vi "VI Tree.vi"   [LabVIEW 2011, in "Agilent PSG MXG Series.lvlib"]
doc: "This is the instrument driver for the Agilent PSG MXG Series. The VI Tree displays all the user-callable VIs of the instrument driver in an organized table."
uses:
  Agilent PSG MXG Series.lvlib
  Configure/Configure Sweep (List).vi
  Configure/Modulation/Configure Modulation (Amplitude).vi
  Configure/Modulation/Configure Modulation Waveform (Noise).vi
panel:
  # "(c) 2011 National Instruments.  ALL RIGHTS RESERVED."
  # "SEE DIAGRAM\nFOR VI TREE."
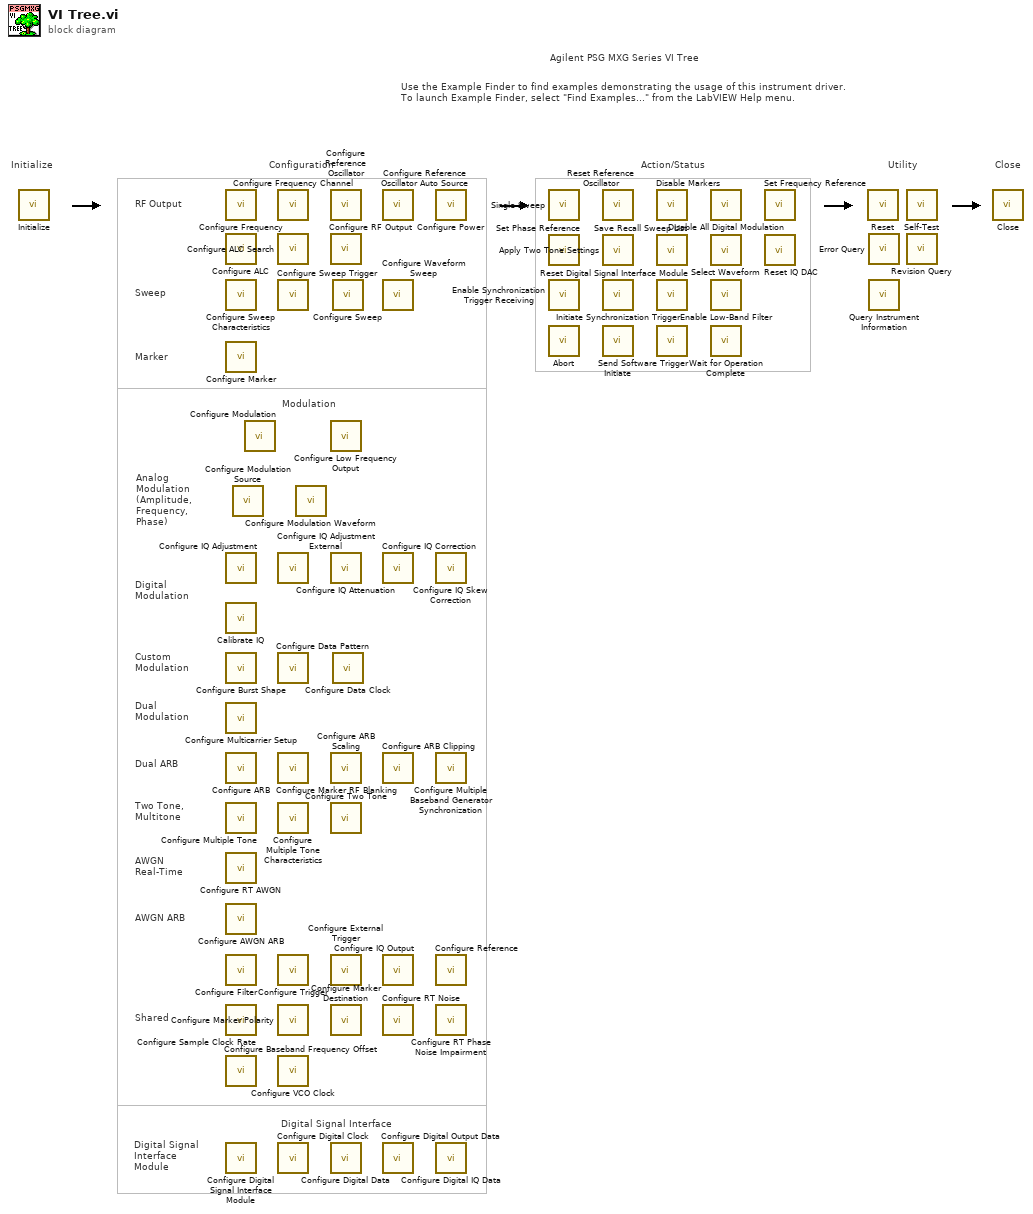
[diagram p0: block diagram]
diagram:
  # "AWGN ARB"
  # "Digital Signal Interface"
  # "Marker"
  # "Digital Signal\nInterface\nModule"
  # "AWGN\nReal-Time"
  # "Shared"
  # "Two Tone,\nMultitone"
  # "Dual ARB"
  # "Dual\nModulation"
  # "Custom\nModulation"
  # "Digital\nModulation"
  # "Analog\nModulation\n(Amplitude,\nFrequency,\nPhase)"
  # "Sweep"
  # "RF Output"
  # "Modulation"
  # "Agilent PSG MXG Series VI Tree"
  # "Use the Example Finder to find examples demonstrating the usage of this instrument driver.\nTo launch Example Finder, select \"Find Examples...\" from the LabVIEW Help menu."
  # "Configuration"
  # "Utility"
  # "Action/Status"
  # "Close"
  # "Initialize"
  n1 = call "Initialize.vi"() -> ()  [unwired: 10 in, 2 out]
  n2 = call "Configure Frequency.vi"() -> ()  [unwired: 14 in, 2 out]
  n3 = call "Configure ALC.vi"() -> ()  [unwired: 14 in, 2 out]
  n4 = call "Configure Sweep Characteristics.vi"() -> ()  [unwired: 14 in, 2 out]
  n5 = call "Configure Marker.vi"() -> ()  [unwired: 14 in, 2 out]
  n6 = call "Configure IQ Adjustment.vi"() -> ()  [unwired: 14 in, 2 out]
  n7 = call "Calibrate IQ.vi"() -> ()  [unwired: 10 in, 2 out]
  n8 = call "Configure Burst Shape.vi"() -> ()  [unwired: 14 in, 2 out]
  n9 = call "Configure Multicarrier Setup.vi"() -> ()  [unwired: 14 in, 2 out]
  n10 = call "Configure ARB.vi"() -> ()  [unwired: 10 in, 2 out]
  n11 = call "Configure Multiple Tone.vi"() -> ()  [unwired: 14 in, 2 out]
  n12 = call "Configure RT AWGN.vi"() -> ()  [unwired: 10 in, 2 out]
  n13 = call "Configure AWGN ARB.vi"() -> ()  [unwired: 10 in, 2 out]
  n14 = call "Configure Filter.vi"() -> ()  [unwired: 14 in, 2 out]
  n15 = call "Configure Sample Clock Rate.vi"() -> ()  [unwired: 10 in, 2 out]
  n16 = call "Configure Baseband Frequency Offset.vi"() -> ()  [unwired: 10 in, 2 out]
  n17 = call "Configure Digital Signal Interface Module.vi"() -> ()  [unwired: 10 in, 2 out]
  n18 = call "Configure Modulation Source.vi"() -> ()  [unwired: 14 in, 2 out]
  n19 = call-poly "Configure Modulation.vi"() -> ()  [unwired: 14 in, 2 out]
  n20 = call "Configure Frequency Channel.vi"() -> ()  [unwired: 10 in, 2 out]
  n21 = call "Configure ALC Search.vi"() -> ()  [unwired: 14 in, 2 out]
  n22 = call "Configure Sweep Trigger.vi"() -> ()  [unwired: 14 in, 2 out]
  n23 = call "Configure IQ Adjustment External.vi"() -> ()  [unwired: 14 in, 2 out]
  n24 = call "Configure Data Pattern.vi"() -> ()  [unwired: 10 in, 2 out]
  n25 = call "Configure Marker RF Blanking.vi"() -> ()  [unwired: 10 in, 2 out]
  n26 = call "Configure Multiple Tone Characteristics.vi"() -> ()  [unwired: 10 in, 2 out]
  n27 = call "Configure Trigger.vi"() -> ()  [unwired: 14 in, 2 out]
  n28 = call "Configure Marker Polarity.vi"() -> ()  [unwired: 10 in, 2 out]
  n29 = call "Configure VCO Clock.vi"() -> ()  [unwired: 10 in, 2 out]
  n30 = call "Configure Digital Clock.vi"() -> ()  [unwired: 14 in, 2 out]
  n31 = call-poly "Configure Modulation Waveform.vi"() -> ()  [unwired: 10 in, 2 out]
  n32 = call "Configure Reference Oscillator.vi"() -> ()  [unwired: 10 in, 2 out]
  n33 = call "Configure RF Output.vi"() -> ()  [unwired: 10 in, 2 out]
  n34 = call "Configure Low Frequency Output.vi"() -> ()  [unwired: 14 in, 2 out]
  n35 = call "Configure IQ Attenuation.vi"() -> ()  [unwired: 10 in, 2 out]
  n36 = call "Configure ARB Scaling.vi"() -> ()  [unwired: 10 in, 2 out]
  n37 = call "Configure Two Tone.vi"() -> ()  [unwired: 10 in, 2 out]
  n38 = call "Configure External Trigger.vi"() -> ()  [unwired: 10 in, 2 out]
  n39 = call "Configure Marker Destination.vi"() -> ()  [unwired: 10 in, 2 out]
  n40 = call "Configure Digital Data.vi"() -> ()  [unwired: 14 in, 2 out]
  n41 = call-poly "Configure Sweep.vi"() -> ()  [unwired: 14 in, 2 out]
  n42 = call "Configure Data Clock.vi"() -> ()  [unwired: 10 in, 2 out]
  n43 = call "Configure Reference Oscillator Auto Source.vi"() -> ()  [unwired: 10 in, 2 out]
  n44 = call "Configure Waveform Sweep.vi"() -> ()  [unwired: 10 in, 2 out]
  n45 = call "Configure IQ Correction.vi"() -> ()  [unwired: 10 in, 2 out]
  n46 = call "Configure ARB Clipping.vi"() -> ()  [unwired: 10 in, 2 out]
  n47 = call "Configure IQ Output.vi"() -> ()  [unwired: 14 in, 2 out]
  n48 = call "Configure RT Noise.vi"() -> ()  [unwired: 14 in, 2 out]
  n49 = call "Configure Digital Output Data.vi"() -> ()  [unwired: 10 in, 2 out]
  n50 = call "Configure Power.vi"() -> ()  [unwired: 14 in, 2 out]
  n51 = call "Configure IQ Skew Correction.vi"() -> ()  [unwired: 10 in, 2 out]
  n52 = call "Configure Multiple Baseband Generator Synchronization.vi"() -> ()  [unwired: 10 in, 2 out]
  n53 = call "Configure Reference.vi"() -> ()  [unwired: 10 in, 2 out]
  n54 = call "Configure RT Phase Noise Impairment.vi"() -> ()  [unwired: 10 in, 2 out]
  n55 = call "Configure Digital IQ Data.vi"() -> ()  [unwired: 14 in, 2 out]
  n56 = call "Single Sweep.vi"() -> ()  [unwired: 10 in, 2 out]
  n57 = call "Set Phase Reference.vi"() -> ()  [unwired: 10 in, 2 out]
  n58 = call "Enable Synchronization Trigger Receiving.vi"() -> ()  [unwired: 10 in, 2 out]
  n59 = call "Abort.vi"() -> ()  [unwired: 10 in, 2 out]
  n60 = call "Reset Reference Oscillator.vi"() -> ()  [unwired: 10 in, 2 out]
  n61 = call "Apply Two Tone Settings.vi"() -> ()  [unwired: 10 in, 2 out]
  n62 = call "Initiate Synchronization Trigger.vi"() -> ()  [unwired: 10 in, 2 out]
  n63 = call "Initiate.vi"() -> ()  [unwired: 10 in, 2 out]
  n64 = call "Disable Markers.vi"() -> ()  [unwired: 10 in, 2 out]
  n65 = call "Save Recall Sweep List.vi"() -> ()  [unwired: 10 in, 2 out]
  n66 = call "Reset Digital Signal Interface Module.vi"() -> ()  [unwired: 10 in, 2 out]
  n67 = call "Send Software Trigger.vi"() -> ()  [unwired: 10 in, 2 out]
  n68 = call "Disable All Digital Modulation.vi"() -> ()  [unwired: 10 in, 2 out]
  n69 = call "Select Waveform.vi"() -> ()  [unwired: 10 in, 2 out]
  n70 = call "Enable Low-Band Filter.vi"() -> ()  [unwired: 10 in, 2 out]
  n71 = call "Wait for Operation Complete.vi"() -> ()  [unwired: 10 in, 2 out]
  n72 = call "Set Frequency Reference.vi"() -> ()  [unwired: 10 in, 2 out]
  n73 = call "Reset IQ DAC.vi"() -> ()  [unwired: 10 in, 2 out]
  n74 = call "Reset.vi"() -> ()  [unwired: 10 in, 2 out]
  n75 = call "Error Query.vi"() -> ()  [unwired: 8 in, 4 out]
  n76 = call "Query Instrument Information.vi"() -> ()  [unwired: 8 in, 8 out]
  n77 = call "Self-Test.vi"() -> ()  [unwired: 8 in, 4 out]
  n78 = call "Revision Query.vi"() -> ()  [unwired: 8 in, 4 out]
  n79 = call "Close.vi"() -> ()  [unwired: 11 in, 1 out]
